vi "CALIBCATION_IMAGE_THRESHOLD_SET.vi"(5 "COM":bool, 7 "VISA name":refnum<visa-resource-name>, 10 "byPara":T1(ring), 11 "data":u16) -> (3 "return":i32)   [LabVIEW 2016]
panel:
  in  "cmd_std_header_t":T2={"byCmdType"=11, "bySubCmd"=195, "byPara"=0, "byAddr_h"=0, "byAddr_l"=0, "byAddr_ll"=0, "byLen_h"=0, "byLen_l"=0}
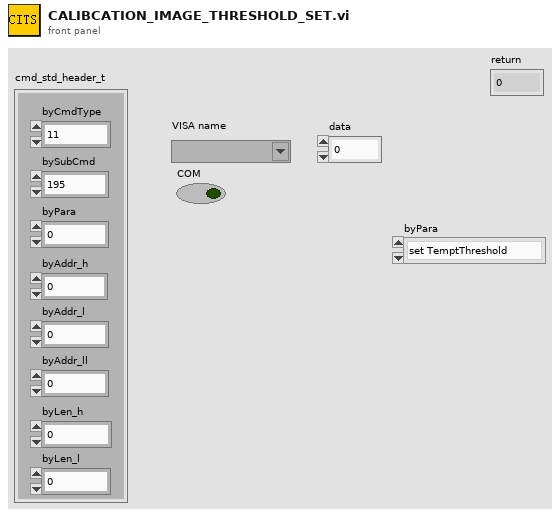
[diagram p1: front panel]
types:
  T1 = enum16{"set TemptThreshold", "set TimeThreshold"}
  T2 = cluster{"byCmdType":u8, "bySubCmd":u8, "byPara":u8, "byAddr_h":u8, "byAddr_l":u8, "byAddr_ll":u8, "byLen_h":u8, "byLen_l":u8}
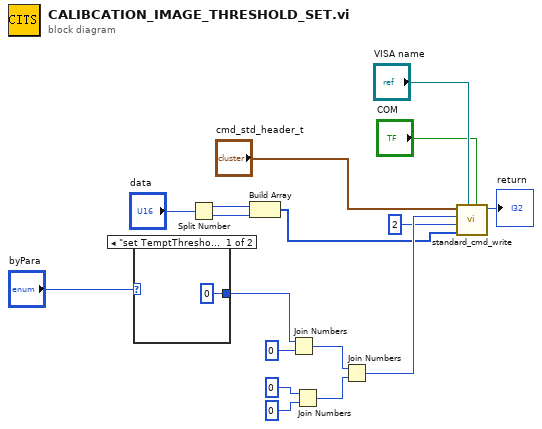
[diagram p0: block diagram]
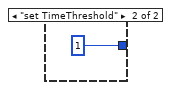
[diagram p2: hidden frame]
diagram:
  n1 = case shown="\"set TemptThreshold\", Default" "byPara" {
    tunnel: [u8 0 u8 1] -> w13
    frame "set TemptThreshold", Default {
    }
    frame "set TimeThreshold" {
    }
  }
  n2 = Split Number(x="data") -> (hi(x)=w4:u8, lo(x)=w3:u8)
  n3 = Build Array(w4, w3) -> (w2:u8[])
  n4 = Join Numbers(hi=w13, lo=u8 0) -> ((hi.lo)=w9:u16)
  n5 = Join Numbers(hi=u8 0, lo=u8 0) -> ((hi.lo)=w8:u16)
  n6 = Join Numbers(hi=w9, lo=w8) -> ((hi.lo)=w7:u32)
  n7 = call "standard_cmd_write.vi"("COM"="COM", "VISA name"="VISA name", "data"=w2, "dwLen"=u32 2, "dwAddr"=w7, "cmd_std_header_t"="cmd_std_header_t") -> ("return"=→"return":i32)  [unwired: 5 in]
